vi "ai_continuous_lite.vi"() -> ()   [LabVIEW 2020]
uses:
  <vilib>/Analysis/baseanly.llb/Mean (DBL).vi
  <vilib>/Analysis/NI_AALBase.lvlib
panel:
  out "数组":dbl[](array[numeric]) format="%.5f"
  out "Rounds":i32
  out "error out":errorcluster caption="错误输出"
  out "AiFifoResidual":i32
  in  "Stop":bool
  out "波形图":sgl[][](graph)
  in  "PointsToRead":u32=10000
  in  "SamplePeriod(ns)":u32=5000
  in  "ChanSel":bool[](array[boolean])=[TRUE, TRUE, TRUE, TRUE, TRUE, TRUE, TRUE, TRUE, FALSE, FALSE, FALSE, FALSE, FALSE, FALSE, FALSE, FALSE, FALSE, FALSE, FALSE, FALSE, FALSE, FALSE, FALSE, FALSE]
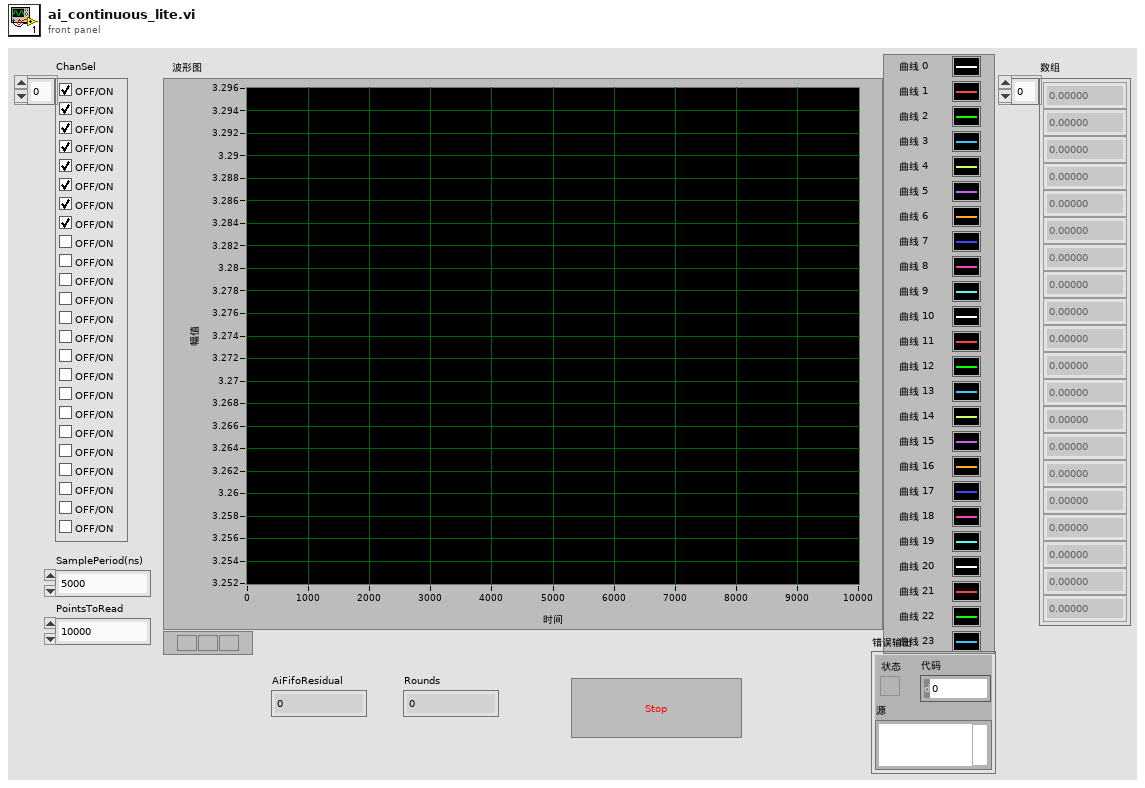
[diagram p1: front panel]
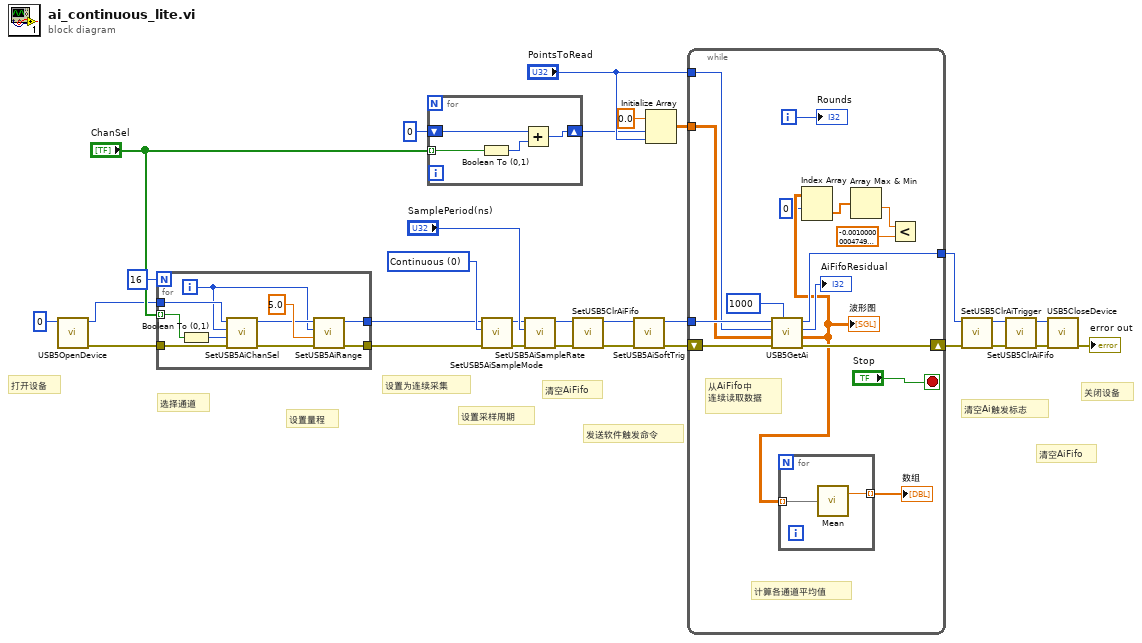
[diagram p0: block diagram]
diagram:
  w27 = u8 0 items=["Continuous", "OneShot"] ("AiSampleMode")
  # "设置量程"
  # "关闭设备"
  # "清空AiFifo"
  # "清空Ai触发标志"
  # "发送软件触发命令"
  # "清空AiFifo"
  # "设置采样周期"
  # "设置为连续采集"
  # "选择通道"
  # "打开设备"
  n1 = call "USB5OpenDevice.vi"("DevIndex"=0) -> ("error out"=w1:errorcluster, "DevIndex Out"=w2:i32)  [unwired: 9 in]
  n2 = for {
    N: 16 -> [_]
    tunnel: w2 -> [w39]
    tunnel: w1 -> [w38]
    tunnel: [w33] -> w5
    tunnel: [w31] -> w4
    tunnel: "ChanSel" -> [w36] mode=indexing
    i -> [w30]
    n3 = Boolean To (0,1)(Boolean=w36) -> (0, 1=w37:i16)
    n4 = call "SetUSB5AiChanSel.vi"("错误输入（无错误）"=w38, "Sel"=w37, "Chan"=w30, "DevIndex"=w39) -> ("错误输出"=w32:errorcluster, "DevIndex Out"=w34:i32)  [unwired: 6 in]
    n5 = call "SetUSB5AiRange.vi"("错误输入（无错误）"=w32, "AiRange"=sgl 5.0, "Chan"=w30, "DevIndex"=w34) -> ("错误输出"=w31:errorcluster, "DevIndex Out"=w33:i32)  [unwired: 6 in]
  }
  n6 = for {
    tunnel: "ChanSel" -> [w43] mode=indexing
    shift-right: [w40] -> w14
    shift-left: i16 0 -> [w41]
    n7 = Boolean To (0,1)(Boolean=w43) -> (0, 1=w42:i16)
    n8 = Add(x=w41, y=w42) -> (x+y=w40:i16)
  }
  n9 = call "SetUSB5AiSampleMode.vi"("错误输入（无错误）"=w4, "AiSampleMode"=w27, "DevIndex"=w5) -> ("错误输出"=w12:errorcluster, "DevIndex Out"=w13:i32)  [unwired: 7 in]
  n10 = call "SetUSB5AiSampleRate.vi"("错误输入（无错误）"=w12, "SamplePeriod(ns)"="SamplePeriod(ns)", "DevIndex"=w13) -> ("错误输出"=w10:errorcluster, "DevIndex Out"=w11:i32)  [unwired: 7 in]
  n11 = call "SetUSB5ClrAiFifo.vi"("错误输入（无错误）"=w10, "DevIndex"=w11) -> ("错误输出"=w25:errorcluster, "DevIndex Out"=w26:i32)  [unwired: 8 in]
  n12 = call "SetUSB5AiSoftTrig.vi"("错误输入（无错误）"=w25, "DevIndex"=w26) -> ("错误输出"=w23:errorcluster, "DevIndex Out"=w24:i32)  [unwired: 8 in]
  n13 = Initialize Array(sgl 0.0 ("元素"), w14, "PointsToRead") -> (w19:sgl[][])
  n14 = while {
    tunnel: w24 -> [w59]
    tunnel: "PointsToRead" -> [w57]
    tunnel: w19 -> [w56]
    tunnel: [w54] -> w6
    shift-right: [w53] -> w9
    shift-left: w23 -> [w58]
    i -> [w52]
    stop <- "Stop" stop-if-true
    # "计算各通道平均值"
    # "从AiFifo中\n连续读取数据"
    n15 = call "USB5GetAi.vi"("TimeOut"=1000, "错误输入（无错误）"=w58, "Ai"=w56, "Points"=w57, "DevIndex"=w59) -> ("错误输出"=w53:errorcluster, "Ai Out"=w47:sgl[][], "AiFifoUsed"=→"AiFifoResidual":i32, "DevIndex Out"=w54:i32)  [unwired: 3 in]
    "波形图" <- w47
    n16 = for {
      tunnel: w47 -> [w61] mode=indexing
      tunnel: [w60] -> w50 mode=indexing
      n17 = call-poly <vilib>:"Mean.vi"("X"=w61) -> ("mean"=w60:dbl)  [unwired: 1 out]
    }
    "数组" <- w50
    n18 = Index Array(array=w47, index (row)=0 ("索引 (行)")) -> (element=w45:sgl[])  [unwired: 1 in]
    n19 = Array Max & Min(array=w45) -> (min value=w49:sgl)  [unwired: 3 out]
    n20 = Less?(x=w49, y=sgl -0.001) -> ()  [unwired: 1 out]
    "Rounds" <- w52
  }
  n21 = call "SetUSB5ClrAiTrigger.vi"("错误输入（无错误）"=w9, "DevIndex"=w6) -> ("错误输出"=w8:errorcluster, "DevIndex Out"=w7:i32)  [unwired: 8 in]
  n22 = call "SetUSB5ClrAiFifo.vi"("错误输入（无错误）"=w8, "DevIndex"=w7) -> ("错误输出"=w18:errorcluster, "DevIndex Out"=w17:i32)  [unwired: 8 in]
  n23 = call "USB5CloseDevice.vi"("错误输入（无错误）"=w18, "DevIndex"=w17) -> ("error out"=→"error out":errorcluster)  [unwired: 8 in, 1 out]
